vi "_PluginLoader_RunPlugins.vi"(8 "error in (no error)":errorcluster, 9 "EventsOut":T1, 11 "_PluginLoader in":refnum<class "_PluginLoader.lvclass">) -> (0 "error out":errorcluster, 3 "_PluginLoader out":refnum<class "_PluginLoader.lvclass">)   [LabVIEW 2014, in "_PluginLoader.lvclass"]
uses:
  _PluginLoader.lvclass
  _LVCMPlugin/GCMPlugin_EventsOut.ctl
  _PluginLoader.lvclass/_PluginLoader.ctl
  GCMPlugin/GCMPlugin.lvclass
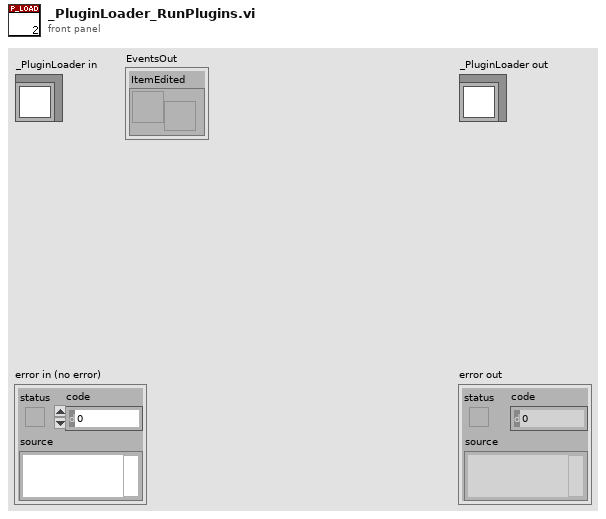
[diagram p1: front panel]
types:
  T1 = typedef "GCMPlugin.lvclass/GCMPlugin_EventsOut.ctl" = cluster{"ItemEdited":refnum<user-event>}
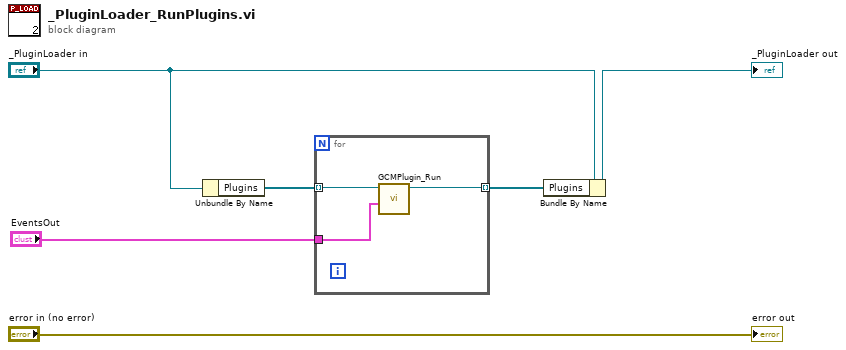
[diagram p0: block diagram]
diagram:
  n1 = Unbundle By Name("_PluginLoader in") -> ("Plugins"=w2:refnum<class "GCMPlugin.lvclass">[])
  n2 = for {
    tunnel: w2 -> [w9] mode=indexing
    tunnel: [w8] -> w1 mode=indexing
    tunnel: "EventsOut" -> [w7]
    n3 = call "GCMPlugin_Run.vi"("EventsOut"=w7, "_LVCMPlugin in"=w9) -> ("_LVCMPlugin out"=w8:refnum<class "GCMPlugin.lvclass">)  [unwired: 8 in, 1 out]
  }
  n4 = Bundle By Name(cluster="_PluginLoader in", "Plugins"=w1) -> (→"_PluginLoader out":refnum<class "_PluginLoader.lvclass">)
  "error out" <- "error in (no error)"
